vi "2D barcode scanning no PSD.vi"() -> ()   [LabVIEW 2017]
panel:
  out "Photodiode 2":dynamicdata(graph)
  in  "All points":bool
  out "Photodiode greater than abs baseline?":bool
  out "Photodiode":dbl
  out "x <= 0?":bool
  out "Vertical Mirror Angle":dynamicdata(graph)
  out "Horizontal Mirror Angle":dynamicdata(graph)
  out "Vertical Angle vs. Photodiode":cluster{"Y":dbl[], "Y":dbl[]}[](graph)
  out "Horizontal Angle vs. Photodiode Falling":cluster{"Y":dbl[], "Y":dbl[]}[](graph)
  out "Horizontal Mirror Driving Voltage":dynamicdata(graph)
  out "Vertical Mirror Driving Voltage":dynamicdata(graph)
  in  "stop (F)":bool
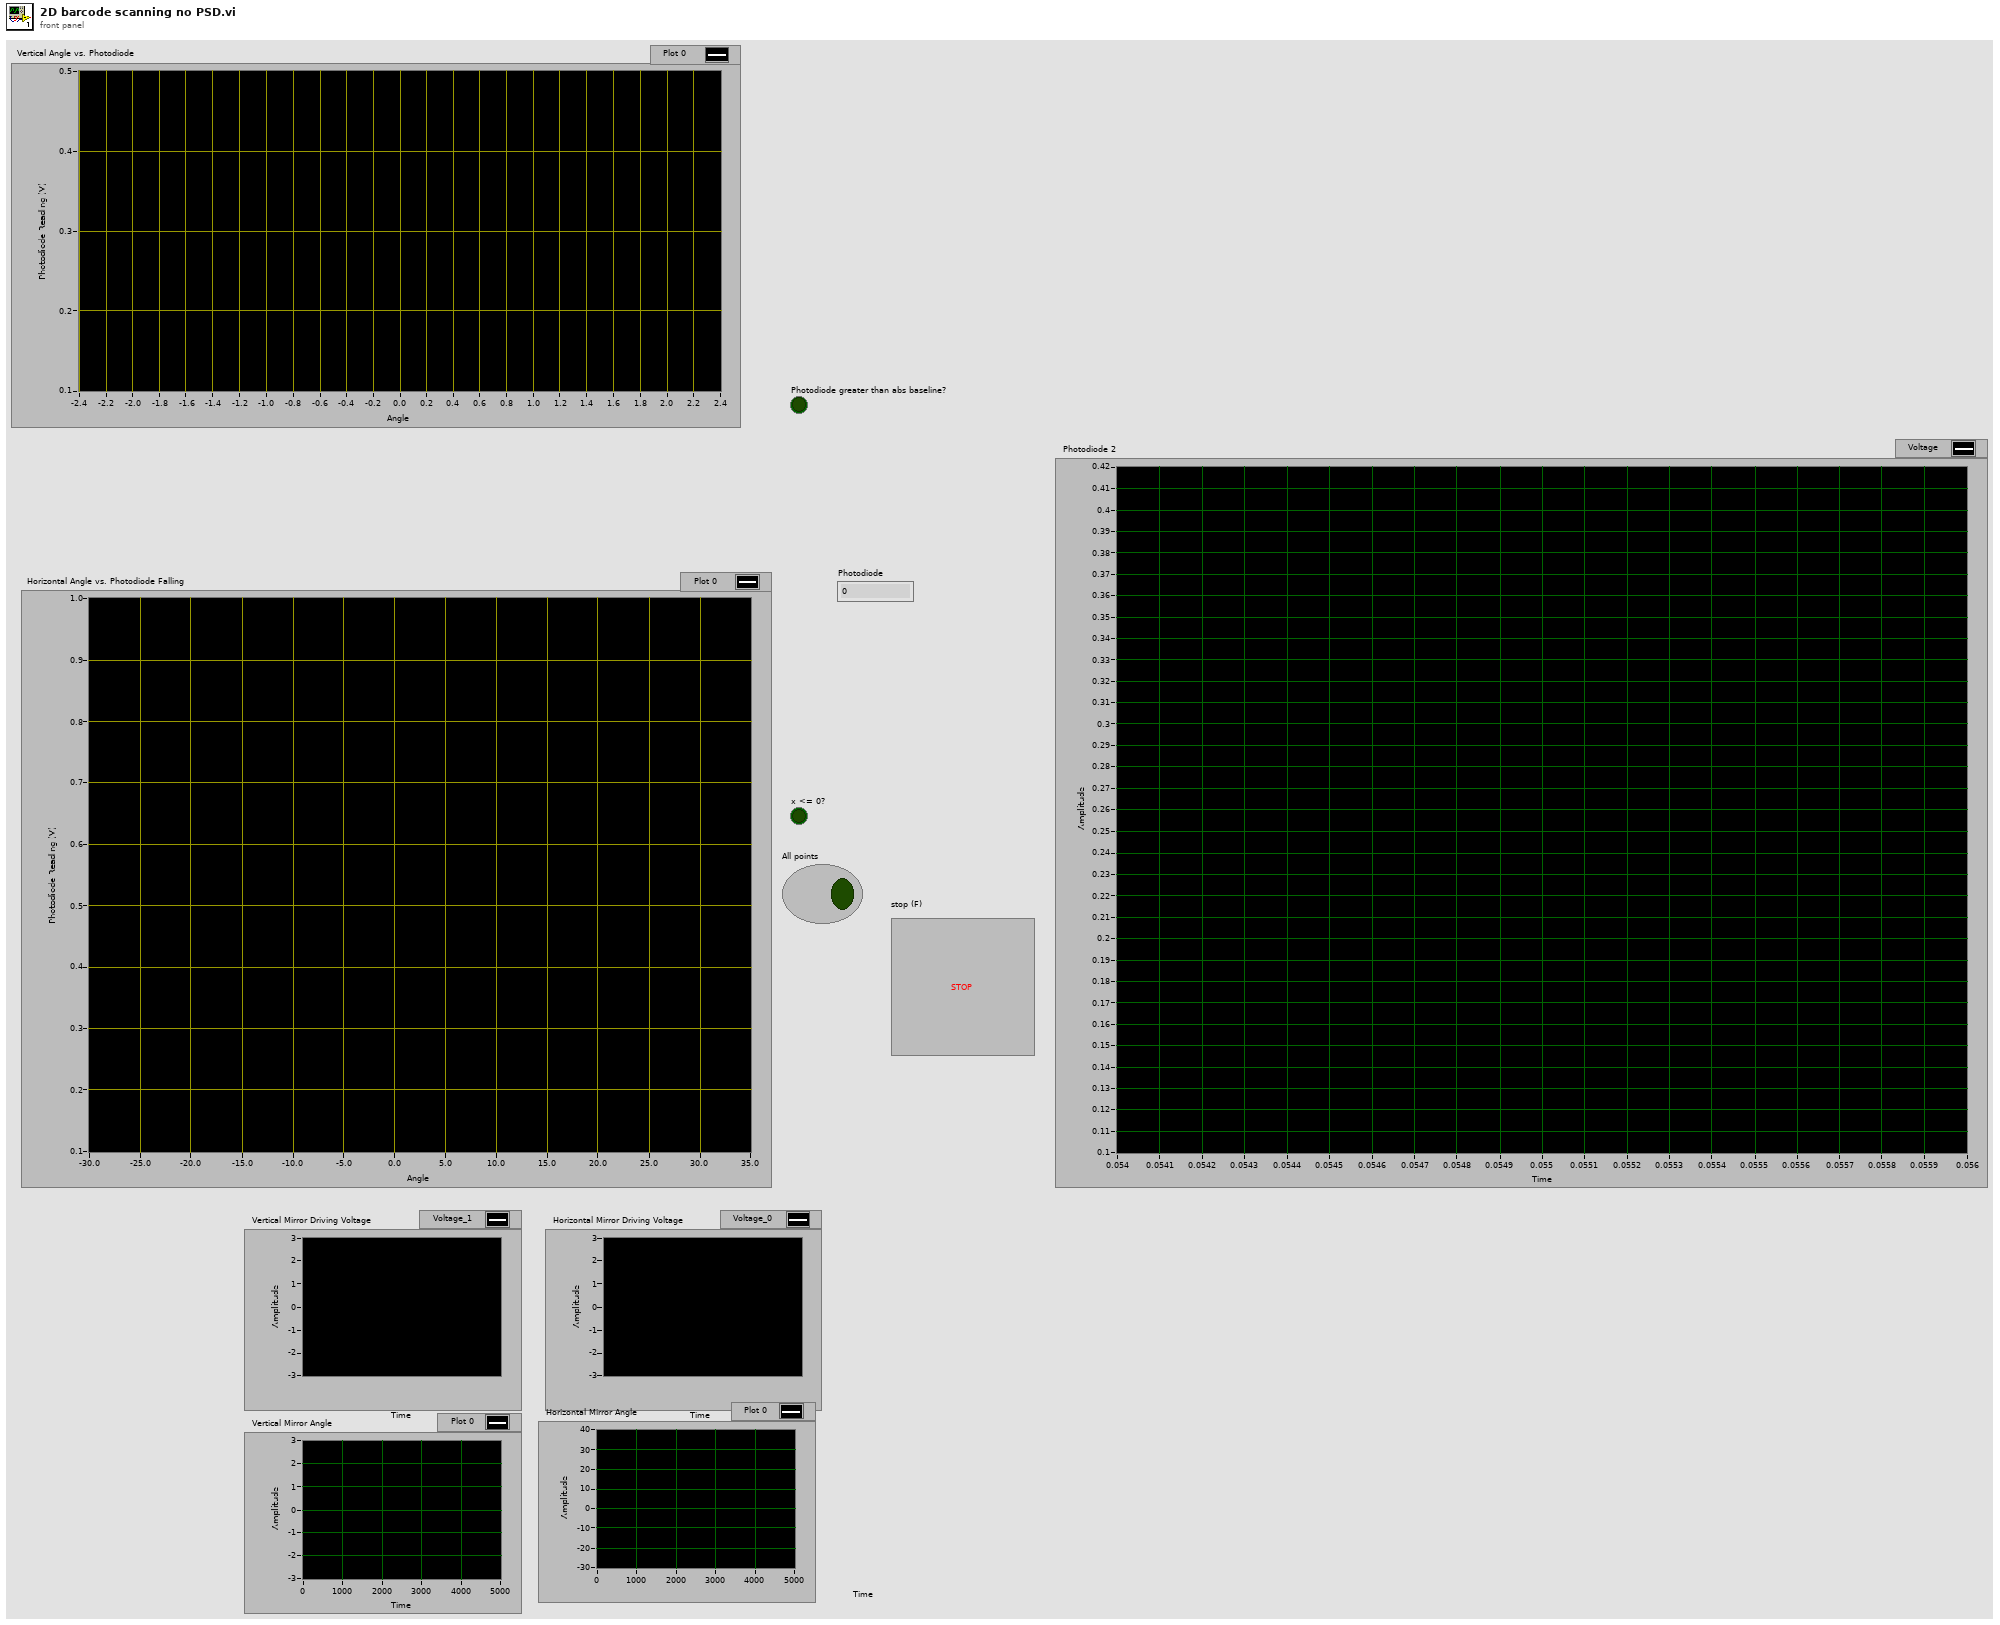
[diagram p1: front panel]
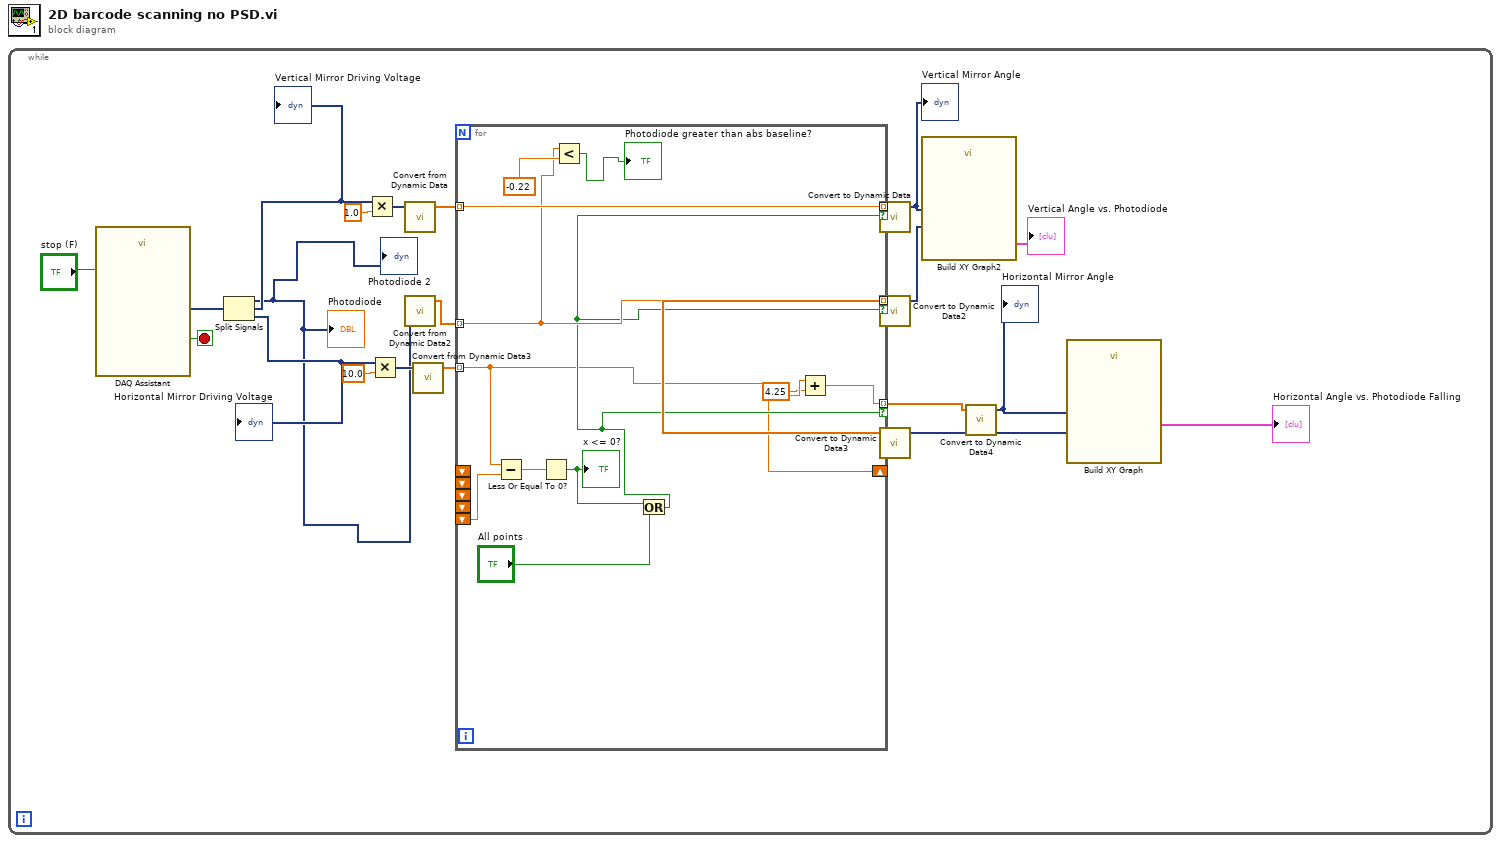
[diagram p0: block diagram]
diagram:
  n1 = while {
    stop <- w21 stop-if-true
    n2 = call "DAQ Assistant"("stop (F)"="stop (F)") -> ("data"=w20:dynamicdata, "stopped"=w21:bool)  [unwired: 15 in, 2 out]
    n3 = Split Signals(w20) -> (w1:dynamicdata, w19:dynamicdata, w2:dynamicdata)  [unwired: 3 in]
    "Vertical Mirror Driving Voltage" <- w19
    "Horizontal Mirror Driving Voltage" <- w2
    "Photodiode" <- w1
    "Photodiode 2" <- w1
    n4 = Multiply(x=w19, y=1.0) -> (x*y=w13:dynamicdata)
    n5 = Multiply(x=w2, y=10.0) -> (x*y=w9:dynamicdata)
    n6 = call "Convert from Dynamic Data"("Dynamic Data Type"=w13) -> ("Array"=w12:dbl[])  [unwired: 3 in]
    n7 = call "Convert from Dynamic Data2"("Dynamic Data Type"=w1) -> ("Array"=w11:dbl[])  [unwired: 3 in]
    n8 = call "Convert from Dynamic Data3"("Dynamic Data Type"=w9) -> ("Array"=w6:dbl[])  [unwired: 3 in]
    n9 = for {
      tunnel: [w34] -> w14 mode=indexing if=w29
      tunnel: w12 -> [w34] mode=indexing
      tunnel: w11 -> [w30] mode=indexing
      tunnel: [w30] -> w5 mode=indexing if=w29
      tunnel: w6 -> [w26] mode=indexing
      tunnel: [w25] -> w3 mode=indexing if=w29
      shift-right: [w26] -> _
      shift-left: _ -> [_]
      shift-left: _ -> [_]
      shift-left: _ -> [_]
      shift-left: _ -> [_]
      shift-left: _ -> [w23]
      n10 = Subtract(x=w26, y=w23) -> (x-y=w33:dbl)
      n11 = Less Or Equal To 0?(x=w33) -> (x <= 0?=w28:bool)
      "x <= 0?" <- w28
      n12 = Less?(x=w30, y=-0.22) -> (x < y?=→"Photodiode greater than abs baseline?":bool)
      n13 = Or(x=w28, y="All points") -> (x .or. y?=w29:bool)
      n14 = Add(x=w26, y=4.25) -> (x+y=w25:dbl)
    }
    n15 = call "Convert to Dynamic Data"("Array"=w14) -> ("Dynamic Data Type"=w8:dynamicdata)  [unwired: 3 in]
    "Vertical Mirror Angle" <- w8
    n16 = call "Convert to Dynamic Data2"("Array"=w5) -> ("Dynamic Data Type"=w10:dynamicdata)  [unwired: 3 in]
    n17 = call "Convert to Dynamic Data3"("Array"=w5) -> ("Dynamic Data Type"=w4:dynamicdata)  [unwired: 3 in]
    n18 = call "Build XY Graph2"("Y Input"=w10, "X Input"=w8) -> ("XY Graph"=→"Vertical Angle vs. Photodiode":cluster{"X":dbl[], "Y":dbl[]}[])  [unwired: 8 in, 1 out]
    n19 = call "Convert to Dynamic Data4"("Array"=w3) -> ("Dynamic Data Type"=w7:dynamicdata)  [unwired: 3 in]
    "Horizontal Mirror Angle" <- w7
    n20 = call "Build XY Graph"("Y Input"=w4, "X Input"=w7) -> ("XY Graph"=→"Horizontal Angle vs. Photodiode Falling":cluster{"X":dbl[], "Y":dbl[]}[])  [unwired: 8 in, 1 out]
  }
